vi "SheetInput (SubVI).vi"(8 "error in (no error)":errorcluster, 11 "The Path to save excel":path=path "E:/程序完善/油菜/side_features") -> (0 "error out":errorcluster, 3 "Cluster":T1)   [LabVIEW 2015]
uses:
  <vilib>/Utility/NIReport.llb/NI_report.lvclass
  <vilib>/addons/_office/_exclsub.llb/font.ctl
  <vilib>/addons/_office/NI_ReportGenerationToolkit.lvlib
  <vilib>/Utility/NIReport.llb/Excel/NI_Excel.lvclass
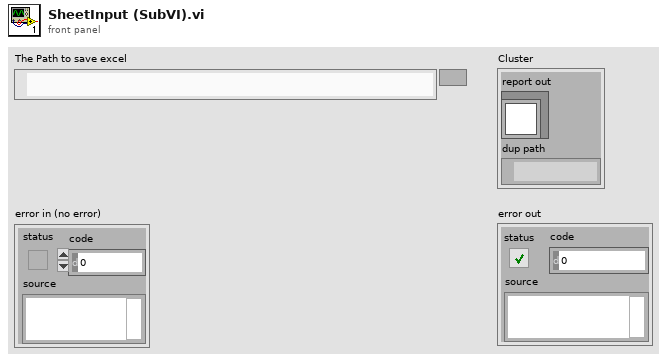
[diagram p1: front panel]
types:
  T1 = cluster{"report out":refnum<class "NI_report.lvclass">, "dup path":path}
  T2 = enum16{"maximized", "minimized", "normal", "no change"}
  T3 = typedef "NI_ReportGenerationToolkit.lvlib/font.ctl" = cluster{"font name":string, "font size":dbl, "bold":u16, "italic":u16, "underline":u16, "strike through":u16, "font color":u32}
  T4 = enum16{"Standard Report", "HTML", "Word", "Excel"}
diagram:
  w407 = T3 {"font name"="", "font size"=13.0, "bold"=0, "italic"=0, "underline"=0, "strike through"=0, "font color"=16777216} ("font")
  w105 = 0 ("column")
  n1 = call <vilib>:"New Report.vi"("window state (normal)"=T2."normal", "report type"=T4."Excel", "error in (no error)"="error in (no error)") -> ("report out"=w9:refnum<class "NI_report.lvclass">, "error out"=w6:errorcluster)  [unwired: 3 in, 8 out]
  n2 = call <vilib>:"Excel Easy Title.vi"("report in"=w9, "title"="Side Features", "start (0, 0)"=cluster{"row":i32, "column":i32} {"row"=0, "column"=0}, "font"=T3 {"font name"="", "font size"=16.0, "bold"=1, "italic"=2, "underline"=2, "strike through"=2, "font color"=0}, "error in (no error)"=w6) -> ("report out"=w106:refnum<class "NI_report.lvclass">, "error out"=w109:errorcluster)  [unwired: 1 in, 8 out]
  n3 = Bundle("row"=1, "column"=w105) -> (w108:cluster{"row":i32, "column":i32})  [unwired: 1 out]
  n4 = Increment(x=w105) -> (x+1=w44:i32)
  n5 = call <vilib>:"Excel Easy Text.vi"("report in"=w106, "border? (F)"=FALSE, "font"=w407, "text"="Serial number", "start (-1, -1)"=w108, "error in (no error)"=w109) -> ("report out"=w55:refnum<class "NI_report.lvclass">, "error out"=w42:errorcluster)  [unwired: 2 in, 6 out]
  n6 = Bundle("row"=1, w44) -> (w59:cluster{"row":i32, i32})  [unwired: 1 out]
  n7 = Increment(x=w44) -> (x+1=w43:i32)
  n8 = call <vilib>:"Excel Easy Text.vi"("report in"=w55, "border? (F)"=FALSE, "font"=w407, "text"="M_TEX_SV", "start (-1, -1)"=w59, "error in (no error)"=w42) -> ("report out"=w46:refnum<class "NI_report.lvclass">, "error out"=w41:errorcluster)  [unwired: 2 in, 6 out]
  n9 = Bundle("row"=1, w43) -> (w51:cluster{"row":i32, i32})  [unwired: 1 out]
  n10 = Increment(x=w43) -> (x+1=w19:i32)
  n11 = call <vilib>:"Excel Easy Text.vi"("report in"=w46, "border? (F)"=FALSE, "font"=w407, "text"="SE_TEX_SV", "start (-1, -1)"=w51, "error in (no error)"=w41) -> ("report out"=w45:refnum<class "NI_report.lvclass">, "error out"=w40:errorcluster)  [unwired: 2 in, 6 out]
  n12 = Bundle("row"=1, w19) -> (w50:cluster{"row":i32, i32})  [unwired: 1 out]
  n13 = Increment(x=w19) -> (x+1=w25:i32)
  n14 = call <vilib>:"Excel Easy Text.vi"("report in"=w45, "border? (F)"=FALSE, "font"=w407, "text"="S_TEX_SV", "start (-1, -1)"=w50, "error in (no error)"=w40) -> ("report out"=w20:refnum<class "NI_report.lvclass">, "error out"=w21:errorcluster)  [unwired: 2 in, 6 out]
  n15 = Bundle("row"=1, w25) -> (w39:cluster{"row":i32, i32})  [unwired: 1 out]
  n16 = Increment(x=w25) -> (x+1=w24:i32)
  n17 = call <vilib>:"Excel Easy Text.vi"("report in"=w20, "border? (F)"=FALSE, "font"=w407, "text"="MU3_TEX_SV", "start (-1, -1)"=w39, "error in (no error)"=w21) -> ("report out"=w27:refnum<class "NI_report.lvclass">, "error out"=w23:errorcluster)  [unwired: 2 in, 6 out]
  n18 = Bundle("row"=1, w24) -> (w32:cluster{"row":i32, i32})  [unwired: 1 out]
  n19 = Increment(x=w24) -> (x+1=w12:i32)
  n20 = call <vilib>:"Excel Easy Text.vi"("report in"=w27, "border? (F)"=FALSE, "font"=w407, "text"="U_TEX_SV", "start (-1, -1)"=w32, "error in (no error)"=w23) -> ("report out"=w26:refnum<class "NI_report.lvclass">, "error out"=w22:errorcluster)  [unwired: 2 in, 6 out]
  n21 = Bundle("row"=1, w12) -> (w31:cluster{"row":i32, i32})  [unwired: 1 out]
  n22 = Increment(x=w12) -> (x+1=w74:i32)
  n23 = call <vilib>:"Excel Easy Text.vi"("report in"=w26, "border? (F)"=FALSE, "font"=w407, "text"="E_TEX_SV", "start (-1, -1)"=w31, "error in (no error)"=w22) -> ("report out"=w14:refnum<class "NI_report.lvclass">, "error out"=w13:errorcluster)  [unwired: 2 in, 6 out]
  n24 = Bundle("row"=1, w74) -> (w15:cluster{"row":i32, i32})  [unwired: 1 out]
  n25 = Increment(x=w74) -> (x+1=w77:i32)
  n26 = call <vilib>:"Excel Easy Text.vi"("report in"=w14, "border? (F)"=FALSE, "font"=w407, "text"="TPA_SV", "start (-1, -1)"=w15, "error in (no error)"=w13) -> ("report out"=w72:refnum<class "NI_report.lvclass">, "error out"=w73:errorcluster)  [unwired: 2 in, 6 out]
  n27 = Bundle("row"=1, w77) -> (w68:cluster{"row":i32, i32})  [unwired: 1 out]
  n28 = Increment(x=w77) -> (x+1=w80:i32)
  n29 = call <vilib>:"Excel Easy Text.vi"("report in"=w72, "border? (F)"=FALSE, "font"=w407, "text"="H_SV", "start (-1, -1)"=w68, "error in (no error)"=w73) -> ("report out"=w75:refnum<class "NI_report.lvclass">, "error out"=w76:errorcluster)  [unwired: 2 in, 6 out]
  n30 = Bundle("row"=1, w80) -> (w60:cluster{"row":i32, i32})  [unwired: 1 out]
  n31 = Increment(x=w80) -> (x+1=w87:i32)
  n32 = call <vilib>:"Excel Easy Text.vi"("report in"=w75, "border? (F)"=FALSE, "font"=w407, "text"="W_SV", "start (-1, -1)"=w60, "error in (no error)"=w76) -> ("report out"=w78:refnum<class "NI_report.lvclass">, "error out"=w79:errorcluster)  [unwired: 2 in, 6 out]
  n33 = Bundle("row"=1, w87) -> (w64:cluster{"row":i32, i32})  [unwired: 1 out]
  n34 = Increment(x=w87) -> (x+1=w94:i32)
  n35 = call <vilib>:"Excel Easy Text.vi"("report in"=w78, "border? (F)"=FALSE, "font"=w407, "text"="HWR_SV", "start (-1, -1)"=w64, "error in (no error)"=w79) -> ("report out"=w85:refnum<class "NI_report.lvclass">, "error out"=w86:errorcluster)  [unwired: 2 in, 6 out]
  n36 = Bundle("row"=1, w94) -> (w81:cluster{"row":i32, i32})  [unwired: 1 out]
  n37 = Increment(x=w94) -> (x+1=w101:i32)
  n38 = call <vilib>:"Excel Easy Text.vi"("report in"=w85, "border? (F)"=FALSE, "font"=w407, "text"="FDNIC_SV", "start (-1, -1)"=w81, "error in (no error)"=w86) -> ("report out"=w92:refnum<class "NI_report.lvclass">, "error out"=w93:errorcluster)  [unwired: 2 in, 6 out]
  n39 = Bundle("row"=1, w101) -> (w88:cluster{"row":i32, i32})  [unwired: 1 out]
  n40 = Increment(x=w101) -> (x+1=w103:i32)
  n41 = call <vilib>:"Excel Easy Text.vi"("report in"=w92, "border? (F)"=FALSE, "font"=w407, "text"="FDIC_SV", "start (-1, -1)"=w88, "error in (no error)"=w93) -> ("report out"=w99:refnum<class "NI_report.lvclass">, "error out"=w100:errorcluster)  [unwired: 2 in, 6 out]
  n42 = Bundle("row"=1, w103) -> (w95:cluster{"row":i32, i32})  [unwired: 1 out]
  n43 = Increment(x=w103) -> (x+1=w150:i32)
  n44 = call <vilib>:"Excel Easy Text.vi"("report in"=w99, "border? (F)"=FALSE, "font"=w407, "text"="R_SV", "start (-1, -1)"=w95, "error in (no error)"=w100) -> ("report out"=w149:refnum<class "NI_report.lvclass">, "error out"=w151:errorcluster)  [unwired: 2 in, 6 out]
  n45 = Bundle("row"=1, w150) -> (w148:cluster{"row":i32, i32})  [unwired: 1 out]
  n46 = Increment(x=w150) -> (x+1=w124:i32)
  n47 = call <vilib>:"Excel Easy Text.vi"("report in"=w149, "border? (F)"=FALSE, "font"=w407, "text"="PAR_SV", "start (-1, -1)"=w148, "error in (no error)"=w151) -> ("report out"=w120:refnum<class "NI_report.lvclass">, "error out"=w121:errorcluster)  [unwired: 2 in, 6 out]
  n48 = Bundle("row"=1, w124) -> (w110:cluster{"row":i32, i32})  [unwired: 1 out]
  n49 = Increment(x=w124) -> (x+1=w131:i32)
  n50 = call <vilib>:"Excel Easy Text.vi"("report in"=w120, "border? (F)"=FALSE, "font"=w407, "text"="HA_SV", "start (-1, -1)"=w110, "error in (no error)"=w121) -> ("report out"=w122:refnum<class "NI_report.lvclass">, "error out"=w123:errorcluster)  [unwired: 2 in, 6 out]
  n51 = Bundle("row"=1, w131) -> (w114:cluster{"row":i32, i32})  [unwired: 1 out]
  n52 = Increment(x=w131) -> (x+1=w138:i32)
  n53 = call <vilib>:"Excel Easy Text.vi"("report in"=w122, "border? (F)"=FALSE, "font"=w407, "text"="AC_SV", "start (-1, -1)"=w114, "error in (no error)"=w123) -> ("report out"=w129:refnum<class "NI_report.lvclass">, "error out"=w130:errorcluster)  [unwired: 2 in, 6 out]
  n54 = Bundle("row"=1, w138) -> (w125:cluster{"row":i32, i32})  [unwired: 1 out]
  n55 = Increment(x=w138) -> (x+1=w145:i32)
  n56 = call <vilib>:"Excel Easy Text.vi"("report in"=w129, "border? (F)"=FALSE, "font"=w407, "text"="M_TEX_SV_FL", "start (-1, -1)"=w125, "error in (no error)"=w130) -> ("report out"=w136:refnum<class "NI_report.lvclass">, "error out"=w137:errorcluster)  [unwired: 2 in, 6 out]
  n57 = Bundle("row"=1, w145) -> (w132:cluster{"row":i32, i32})  [unwired: 1 out]
  n58 = Increment(x=w145) -> (x+1=w147:i32)
  n59 = call <vilib>:"Excel Easy Text.vi"("report in"=w136, "border? (F)"=FALSE, "font"=w407, "text"="SE_TEX_SV_FL", "start (-1, -1)"=w132, "error in (no error)"=w137) -> ("report out"=w143:refnum<class "NI_report.lvclass">, "error out"=w144:errorcluster)  [unwired: 2 in, 6 out]
  n60 = Bundle("row"=1, w147) -> (w139:cluster{"row":i32, i32})  [unwired: 1 out]
  n61 = Increment(x=w147) -> (x+1=w218:i32)
  n62 = call <vilib>:"Excel Easy Text.vi"("report in"=w143, "border? (F)"=FALSE, "font"=w407, "text"="S_TEX_SV_FL", "start (-1, -1)"=w139, "error in (no error)"=w144) -> ("report out"=w220:refnum<class "NI_report.lvclass">, "error out"=w221:errorcluster)  [unwired: 2 in, 6 out]
  n63 = Bundle("row"=1, w218) -> (w219:cluster{"row":i32, i32})  [unwired: 1 out]
  n64 = Increment(x=w218) -> (x+1=w166:i32)
  n65 = call <vilib>:"Excel Easy Text.vi"("report in"=w220, "border? (F)"=FALSE, "font"=w407, "text"="MU3_TEX_SV_FL", "start (-1, -1)"=w219, "error in (no error)"=w221) -> ("report out"=w158:refnum<class "NI_report.lvclass">, "error out"=w159:errorcluster)  [unwired: 2 in, 6 out]
  n66 = Bundle("row"=1, w166) -> (w154:cluster{"row":i32, i32})  [unwired: 1 out]
  n67 = Increment(x=w166) -> (x+1=w173:i32)
  n68 = call <vilib>:"Excel Easy Text.vi"("report in"=w158, "border? (F)"=FALSE, "font"=w407, "text"="U_TEX_SV_FL", "start (-1, -1)"=w154, "error in (no error)"=w159) -> ("report out"=w164:refnum<class "NI_report.lvclass">, "error out"=w165:errorcluster)  [unwired: 2 in, 6 out]
  n69 = Bundle("row"=1, w173) -> (w160:cluster{"row":i32, i32})  [unwired: 1 out]
  n70 = Increment(x=w173) -> (x+1=w175:i32)
  n71 = call <vilib>:"Excel Easy Text.vi"("report in"=w164, "border? (F)"=FALSE, "font"=w407, "text"="E_TEX_SV_FL", "start (-1, -1)"=w160, "error in (no error)"=w165) -> ("report out"=w171:refnum<class "NI_report.lvclass">, "error out"=w172:errorcluster)  [unwired: 2 in, 6 out]
  n72 = Bundle("row"=1, w175) -> (w167:cluster{"row":i32, i32})  [unwired: 1 out]
  n73 = Increment(x=w175) -> (x+1=w216:i32)
  n74 = call <vilib>:"Excel Easy Text.vi"("report in"=w171, "border? (F)"=FALSE, "font"=w407, "text"="YPA_SV_FL", "start (-1, -1)"=w167, "error in (no error)"=w172) -> ("report out"=w215:refnum<class "NI_report.lvclass">, "error out"=w217:errorcluster)  [unwired: 2 in, 6 out]
  n75 = Bundle("row"=1, w216) -> (w214:cluster{"row":i32, i32})  [unwired: 1 out]
  n76 = Increment(x=w216) -> (x+1=w190:i32)
  n77 = call <vilib>:"Excel Easy Text.vi"("report in"=w215, "border? (F)"=FALSE, "font"=w407, "text"="H_SV_FL", "start (-1, -1)"=w214, "error in (no error)"=w217) -> ("report out"=w186:refnum<class "NI_report.lvclass">, "error out"=w187:errorcluster)  [unwired: 2 in, 6 out]
  n78 = Bundle("row"=1, w190) -> (w176:cluster{"row":i32, i32})  [unwired: 1 out]
  n79 = Increment(x=w190) -> (x+1=w197:i32)
  n80 = call <vilib>:"Excel Easy Text.vi"("report in"=w186, "border? (F)"=FALSE, "font"=w407, "text"="W_SV_FL", "start (-1, -1)"=w176, "error in (no error)"=w187) -> ("report out"=w188:refnum<class "NI_report.lvclass">, "error out"=w189:errorcluster)  [unwired: 2 in, 6 out]
  n81 = Bundle("row"=1, w197) -> (w180:cluster{"row":i32, i32})  [unwired: 1 out]
  n82 = Increment(x=w197) -> (x+1=w204:i32)
  n83 = call <vilib>:"Excel Easy Text.vi"("report in"=w188, "border? (F)"=FALSE, "font"=w407, "text"="HWR_SV_FL", "start (-1, -1)"=w180, "error in (no error)"=w189) -> ("report out"=w195:refnum<class "NI_report.lvclass">, "error out"=w196:errorcluster)  [unwired: 2 in, 6 out]
  n84 = Bundle("row"=1, w204) -> (w191:cluster{"row":i32, i32})  [unwired: 1 out]
  n85 = Increment(x=w204) -> (x+1=w211:i32)
  n86 = call <vilib>:"Excel Easy Text.vi"("report in"=w195, "border? (F)"=FALSE, "font"=w407, "text"="FDNIC_SV_FL", "start (-1, -1)"=w191, "error in (no error)"=w196) -> ("report out"=w202:refnum<class "NI_report.lvclass">, "error out"=w203:errorcluster)  [unwired: 2 in, 6 out]
  n87 = Bundle("row"=1, w211) -> (w198:cluster{"row":i32, i32})  [unwired: 1 out]
  n88 = Increment(x=w211) -> (x+1=w213:i32)
  n89 = call <vilib>:"Excel Easy Text.vi"("report in"=w202, "border? (F)"=FALSE, "font"=w407, "text"="FDIC_SV_FL", "start (-1, -1)"=w198, "error in (no error)"=w203) -> ("report out"=w209:refnum<class "NI_report.lvclass">, "error out"=w210:errorcluster)  [unwired: 2 in, 6 out]
  n90 = Bundle("row"=1, w213) -> (w205:cluster{"row":i32, i32})  [unwired: 1 out]
  n91 = Increment(x=w213) -> (x+1=w337:i32)
  n92 = call <vilib>:"Excel Easy Text.vi"("report in"=w209, "border? (F)"=FALSE, "font"=w407, "text"="R_SV_FL", "start (-1, -1)"=w205, "error in (no error)"=w210) -> ("report out"=w338:refnum<class "NI_report.lvclass">, "error out"=w339:errorcluster)  [unwired: 2 in, 6 out]
  n93 = Bundle("row"=1, w337) -> (w340:cluster{"row":i32, i32})  [unwired: 1 out]
  n94 = Increment(x=w337) -> (x+1=w265:i32)
  n95 = call <vilib>:"Excel Easy Text.vi"("report in"=w338, "border? (F)"=FALSE, "font"=w407, "text"="PAR_SV_FL", "start (-1, -1)"=w340, "error in (no error)"=w339) -> ("report out"=w264:refnum<class "NI_report.lvclass">, "error out"=w266:errorcluster)  [unwired: 2 in, 6 out]
  n96 = Bundle("row"=1, w265) -> (w263:cluster{"row":i32, i32})  [unwired: 1 out]
  n97 = Increment(x=w265) -> (x+1=w239:i32)
  n98 = call <vilib>:"Excel Easy Text.vi"("report in"=w264, "border? (F)"=FALSE, "font"=w407, "text"="HA_SV_FL", "start (-1, -1)"=w263, "error in (no error)"=w266) -> ("report out"=w235:refnum<class "NI_report.lvclass">, "error out"=w236:errorcluster)  [unwired: 2 in, 6 out]
  n99 = Bundle("row"=1, w239) -> (w225:cluster{"row":i32, i32})  [unwired: 1 out]
  n100 = Increment(x=w239) -> (x+1=w246:i32)
  n101 = call <vilib>:"Excel Easy Text.vi"("report in"=w235, "border? (F)"=FALSE, "font"=w407, "text"="AC_SV_FL", "start (-1, -1)"=w225, "error in (no error)"=w236) -> ("report out"=w237:refnum<class "NI_report.lvclass">, "error out"=w238:errorcluster)  [unwired: 2 in, 6 out]
  n102 = Bundle("row"=1, w246) -> (w229:cluster{"row":i32, i32})  [unwired: 1 out]
  n103 = Increment(x=w246) -> (x+1=w253:i32)
  n104 = call <vilib>:"Excel Easy Text.vi"("report in"=w237, "border? (F)"=FALSE, "font"=w407, "text"="FN_SV", "start (-1, -1)"=w229, "error in (no error)"=w238) -> ("report out"=w244:refnum<class "NI_report.lvclass">, "error out"=w245:errorcluster)  [unwired: 2 in, 6 out]
  n105 = Bundle("row"=1, w253) -> (w240:cluster{"row":i32, i32})  [unwired: 1 out]
  n106 = Increment(x=w253) -> (x+1=w260:i32)
  n107 = call <vilib>:"Excel Easy Text.vi"("report in"=w244, "border? (F)"=FALSE, "font"=w407, "text"="GPA_SV", "start (-1, -1)"=w240, "error in (no error)"=w245) -> ("report out"=w251:refnum<class "NI_report.lvclass">, "error out"=w252:errorcluster)  [unwired: 2 in, 6 out]
  n108 = Bundle("row"=1, w260) -> (w247:cluster{"row":i32, i32})  [unwired: 1 out]
  n109 = Increment(x=w260) -> (x+1=w262:i32)
  n110 = call <vilib>:"Excel Easy Text.vi"("report in"=w251, "border? (F)"=FALSE, "font"=w407, "text"="GPAR_SV", "start (-1, -1)"=w247, "error in (no error)"=w252) -> ("report out"=w258:refnum<class "NI_report.lvclass">, "error out"=w259:errorcluster)  [unwired: 2 in, 6 out]
  n111 = Bundle("row"=1, w262) -> (w254:cluster{"row":i32, i32})  [unwired: 1 out]
  n112 = Increment(x=w262) -> (x+1=w333:i32)
  n113 = call <vilib>:"Excel Easy Text.vi"("report in"=w258, "border? (F)"=FALSE, "font"=w407, "text"="YPAR_SV", "start (-1, -1)"=w254, "error in (no error)"=w259) -> ("report out"=w335:refnum<class "NI_report.lvclass">, "error out"=w336:errorcluster)  [unwired: 2 in, 6 out]
  n114 = Bundle("row"=1, w333) -> (w334:cluster{"row":i32, i32})  [unwired: 1 out]
  n115 = Increment(x=w333) -> (x+1=w281:i32)
  n116 = call <vilib>:"Excel Easy Text.vi"("report in"=w335, "border? (F)"=FALSE, "font"=w407, "text"="PC1_SV", "start (-1, -1)"=w334, "error in (no error)"=w336) -> ("report out"=w273:refnum<class "NI_report.lvclass">, "error out"=w274:errorcluster)  [unwired: 2 in, 6 out]
  n117 = Bundle("row"=1, w281) -> (w269:cluster{"row":i32, i32})  [unwired: 1 out]
  n118 = Increment(x=w281) -> (x+1=w288:i32)
  n119 = call <vilib>:"Excel Easy Text.vi"("report in"=w273, "border? (F)"=FALSE, "font"=w407, "text"="PC2_SV", "start (-1, -1)"=w269, "error in (no error)"=w274) -> ("report out"=w279:refnum<class "NI_report.lvclass">, "error out"=w280:errorcluster)  [unwired: 2 in, 6 out]
  n120 = Bundle("row"=1, w288) -> (w275:cluster{"row":i32, i32})  [unwired: 1 out]
  n121 = Increment(x=w288) -> (x+1=w290:i32)
  n122 = call <vilib>:"Excel Easy Text.vi"("report in"=w279, "border? (F)"=FALSE, "font"=w407, "text"="PC3_SV", "start (-1, -1)"=w275, "error in (no error)"=w280) -> ("report out"=w286:refnum<class "NI_report.lvclass">, "error out"=w287:errorcluster)  [unwired: 2 in, 6 out]
  n123 = Bundle("row"=1, w290) -> (w282:cluster{"row":i32, i32})  [unwired: 1 out]
  n124 = Increment(x=w290) -> (x+1=w331:i32)
  n125 = call <vilib>:"Excel Easy Text.vi"("report in"=w286, "border? (F)"=FALSE, "font"=w407, "text"="PC4_SV", "start (-1, -1)"=w282, "error in (no error)"=w287) -> ("report out"=w330:refnum<class "NI_report.lvclass">, "error out"=w332:errorcluster)  [unwired: 2 in, 6 out]
  n126 = Bundle("row"=1, w331) -> (w329:cluster{"row":i32, i32})  [unwired: 1 out]
  n127 = Increment(x=w331) -> (x+1=w305:i32)
  n128 = call <vilib>:"Excel Easy Text.vi"("report in"=w330, "border? (F)"=FALSE, "font"=w407, "text"="PC5_SV", "start (-1, -1)"=w329, "error in (no error)"=w332) -> ("report out"=w301:refnum<class "NI_report.lvclass">, "error out"=w302:errorcluster)  [unwired: 2 in, 6 out]
  n129 = Bundle("row"=1, w305) -> (w291:cluster{"row":i32, i32})  [unwired: 1 out]
  n130 = Increment(x=w305) -> (x+1=w312:i32)
  n131 = call <vilib>:"Excel Easy Text.vi"("report in"=w301, "border? (F)"=FALSE, "font"=w407, "text"="PC6_SV", "start (-1, -1)"=w291, "error in (no error)"=w302) -> ("report out"=w303:refnum<class "NI_report.lvclass">, "error out"=w304:errorcluster)  [unwired: 2 in, 6 out]
  n132 = Bundle("row"=1, w312) -> (w295:cluster{"row":i32, i32})  [unwired: 1 out]
  n133 = Increment(x=w312) -> (x+1=w319:i32)
  n134 = call <vilib>:"Excel Easy Text.vi"("report in"=w303, "border? (F)"=FALSE, "font"=w407, "text"="F1", "start (-1, -1)"=w295, "error in (no error)"=w304) -> ("report out"=w310:refnum<class "NI_report.lvclass">, "error out"=w311:errorcluster)  [unwired: 2 in, 6 out]
  n135 = Bundle("row"=1, w319) -> (w306:cluster{"row":i32, i32})  [unwired: 1 out]
  n136 = Increment(x=w319) -> (x+1=w326:i32)
  n137 = call <vilib>:"Excel Easy Text.vi"("report in"=w310, "border? (F)"=FALSE, "font"=w407, "text"="F2", "start (-1, -1)"=w306, "error in (no error)"=w311) -> ("report out"=w317:refnum<class "NI_report.lvclass">, "error out"=w318:errorcluster)  [unwired: 2 in, 6 out]
  n138 = Bundle("row"=1, w326) -> (w313:cluster{"row":i32, i32})  [unwired: 1 out]
  n139 = Increment(x=w326) -> (x+1=w328:i32)
  n140 = call <vilib>:"Excel Easy Text.vi"("report in"=w317, "border? (F)"=FALSE, "font"=w407, "text"="F3", "start (-1, -1)"=w313, "error in (no error)"=w318) -> ("report out"=w324:refnum<class "NI_report.lvclass">, "error out"=w325:errorcluster)  [unwired: 2 in, 6 out]
  n141 = Bundle("row"=1, w328) -> (w320:cluster{"row":i32, i32})  [unwired: 1 out]
  n142 = Increment(x=w328) -> (x+1=w410:i32)
  n143 = call <vilib>:"Excel Easy Text.vi"("report in"=w324, "border? (F)"=FALSE, "font"=w407, "text"="F4", "start (-1, -1)"=w320, "error in (no error)"=w325) -> ("report out"=w409:refnum<class "NI_report.lvclass">, "error out"=w406:errorcluster)  [unwired: 2 in, 6 out]
  n144 = Bundle("row"=1, w410) -> (w408:cluster{"row":i32, i32})  [unwired: 1 out]
  n145 = Increment(x=w410) -> (x+1=w350:i32)
  n146 = call <vilib>:"Excel Easy Text.vi"("report in"=w409, "border? (F)"=FALSE, "font"=w407, "text"="F5", "start (-1, -1)"=w408, "error in (no error)"=w406) -> ("report out"=w347:refnum<class "NI_report.lvclass">, "error out"=w348:errorcluster)  [unwired: 2 in, 6 out]
  n147 = Bundle("row"=1, w350) -> (w343:cluster{"row":i32, i32})  [unwired: 1 out]
  n148 = Increment(x=w350) -> (x+1=w402:i32)
  n149 = call <vilib>:"Excel Easy Text.vi"("report in"=w347, "border? (F)"=FALSE, "font"=w407, "text"="F6", "start (-1, -1)"=w343, "error in (no error)"=w348) -> ("report out"=w404:refnum<class "NI_report.lvclass">, "error out"=w405:errorcluster)  [unwired: 2 in, 6 out]
  n150 = Bundle("row"=1, w402) -> (w403:cluster{"row":i32, i32})  [unwired: 1 out]
  n151 = Increment(x=w402) -> (x+1=w365:i32)
  n152 = call <vilib>:"Excel Easy Text.vi"("report in"=w404, "border? (F)"=FALSE, "font"=w407, "text"="F7", "start (-1, -1)"=w403, "error in (no error)"=w405) -> ("report out"=w357:refnum<class "NI_report.lvclass">, "error out"=w358:errorcluster)  [unwired: 2 in, 6 out]
  n153 = Bundle("row"=1, w365) -> (w353:cluster{"row":i32, i32})  [unwired: 1 out]
  n154 = Increment(x=w365) -> (x+1=w372:i32)
  n155 = call <vilib>:"Excel Easy Text.vi"("report in"=w357, "border? (F)"=FALSE, "font"=w407, "text"="F8", "start (-1, -1)"=w353, "error in (no error)"=w358) -> ("report out"=w363:refnum<class "NI_report.lvclass">, "error out"=w364:errorcluster)  [unwired: 2 in, 6 out]
  n156 = Bundle("row"=1, w372) -> (w359:cluster{"row":i32, i32})  [unwired: 1 out]
  n157 = Increment(x=w372) -> (x+1=w374:i32)
  n158 = call <vilib>:"Excel Easy Text.vi"("report in"=w363, "border? (F)"=FALSE, "font"=w407, "text"="F9", "start (-1, -1)"=w359, "error in (no error)"=w364) -> ("report out"=w370:refnum<class "NI_report.lvclass">, "error out"=w371:errorcluster)  [unwired: 2 in, 6 out]
  n159 = Bundle("row"=1, w374) -> (w366:cluster{"row":i32, i32})  [unwired: 1 out]
  n160 = Increment(x=w374) -> (x+1=w400:i32)
  n161 = call <vilib>:"Excel Easy Text.vi"("report in"=w370, "border? (F)"=FALSE, "font"=w407, "text"="F10", "start (-1, -1)"=w366, "error in (no error)"=w371) -> ("report out"=w399:refnum<class "NI_report.lvclass">, "error out"=w401:errorcluster)  [unwired: 2 in, 6 out]
  n162 = Bundle("row"=1, w400) -> (w398:cluster{"row":i32, i32})  [unwired: 1 out]
  n163 = Increment(x=w400) -> (x+1=w389:i32)
  n164 = call <vilib>:"Check if File or Folder Exists.vi"("path"="The Path to save excel") -> ("error out"=w418:errorcluster, "file or folder exists?"=w416:bool, "dup path"=w417:path)  [unwired: 8 in]
  n165 = case shown="True" w416 {
    tunnel: [w424 w429] -> w420
    tunnel: w417 -> [w424 w425]
    tunnel: w418 -> [_ _]
    frame False {
    }
    frame True {
      n166 = Get Date/Time In Seconds() -> (seconds since 1Jan1904=w431:timestamp)
      n167 = Path To String(path=w425) -> (string=w428:string)
      n168 = Format Date/Time String(time format string (%c)=".xls", seconds (now)=w431) -> (date/time string=w427:string)  [unwired: 1 out]
      n169 = Concatenate Strings(w428, w427) -> (w426:string)
      n170 = String To Path(string=w426) -> (path=w429:path)
    }
  }
  n171 = call <vilib>:"Excel Easy Text.vi"("report in"=w399, "border? (F)"=FALSE, "font"=w407, "text"="F11", "start (-1, -1)"=w398, "error in (no error)"=w401) -> ("report out"=w385:refnum<class "NI_report.lvclass">, "error out"=w386:errorcluster)  [unwired: 2 in, 6 out]
  n172 = Bundle("row"=1, w389) -> (w375:cluster{"row":i32, i32})  [unwired: 1 out]
  n173 = Increment(x=w389) -> (x+1=w396:i32)
  n174 = call <vilib>:"Excel Easy Text.vi"("report in"=w385, "border? (F)"=FALSE, "font"=w407, "text"="F12", "start (-1, -1)"=w375, "error in (no error)"=w386) -> ("report out"=w387:refnum<class "NI_report.lvclass">, "error out"=w388:errorcluster)  [unwired: 2 in, 6 out]
  n175 = Bundle("row"=1, w396) -> (w379:cluster{"row":i32, i32})  [unwired: 1 out]
  n176 = Increment(x=w396) -> (x+1=w397:i32)
  n177 = call <vilib>:"Excel Easy Text.vi"("report in"=w387, "border? (F)"=FALSE, "font"=w407, "text"="F13", "start (-1, -1)"=w379, "error in (no error)"=w388) -> ("report out"=w394:refnum<class "NI_report.lvclass">, "error out"=w395:errorcluster)  [unwired: 2 in, 6 out]
  n178 = Bundle("row"=1, w397) -> (w390:cluster{"row":i32, i32})  [unwired: 1 out]
  n179 = call <vilib>:"Excel Easy Text.vi"("report in"=w394, "border? (F)"=FALSE, "font"=w407, "text"="F14", "start (-1, -1)"=w390, "error in (no error)"=w395) -> ("report out"=w411:refnum<class "NI_report.lvclass">, "error out"=w412:errorcluster)  [unwired: 2 in, 6 out]
  n180 = call <vilib>:"Excel Set Cell Dimension.vi"("report in"=w411, "width (-1)"=1.2, "error in (no error)"=w412) -> ("report out"=w413:refnum<class "NI_report.lvclass">, "error out"=w414:errorcluster)  [unwired: 11 in]
  n181 = call <vilib>:"Excel Get ActiveX References.vi"("report in"=w413, "error in (no error)"=w414) -> ("report out"=w419:refnum<class "NI_report.lvclass">, "Excel._Worksheet"=w2:refnum<k7>, "error out"=w1:errorcluster)  [unwired: 7 in, 4 out]
  n182 = Bundle("report out"=w419, "dup path"=w420) -> (→"Cluster":T1)  [unwired: 1 in]
  n183 = property class="_Worksheet" props=["Cells"](reference=w2, error in=w1) -> (error out=→"error out":errorcluster)  [unwired: 2 out]
